vi "Display YAML in Tree.vi"(8 "error in (no error)":errorcluster, 10 "Tree Refnum":refnum<vi>, 11 "YAML Parser in":refnum<class "YAML Parser.lvclass">) -> (0 "error out":errorcluster, 3 "YAML Parser out":refnum<class "YAML Parser.lvclass">)   [LabVIEW 2015, in "YAML Parser.lvclass"]
uses:
  YAML Parser.lvclass
  YAML Parser.lvclass/YAML Parser.ctl
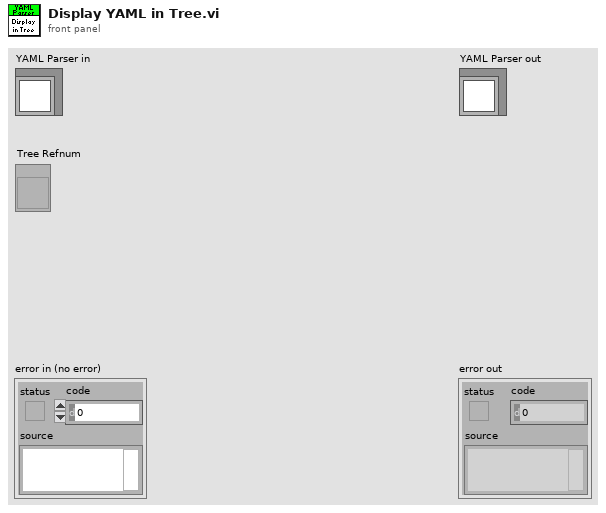
[diagram p1: front panel]
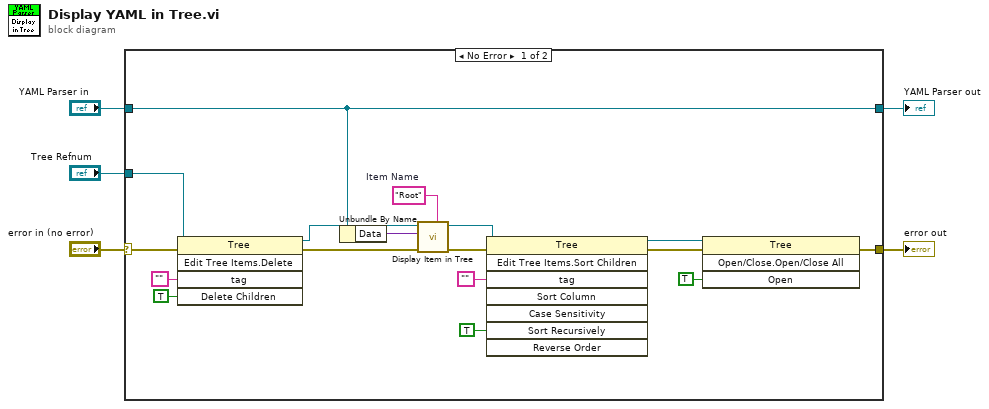
[diagram p0: block diagram]
diagram:
  n1 = case shown="No Error" "error in (no error)" {
    selector: "error in (no error)" -> [w22 w24]
    tunnel: [w11 w24] -> w4
    tunnel: [w18 w23] -> w2
    tunnel: "YAML Parser in" -> [w18 w23]
    tunnel: "Tree Refnum" -> [w21 _]
    frame No Error {
      w8 = "Root"  # Item Name
      n2 = invoke class="Tree" method="Edit Tree Items.Delete"(reference=w21, error in=w22, "tag"="", "Delete Children"=TRUE) -> (reference out=w15:refnum<vi>, error out=w17:errorcluster)  [unwired: 1 in, 3 out]
      n3 = Unbundle By Name(w18) -> ("Data"=w16:variant)
      n4 = call "Display Item in Tree.vi"("Item Name"=w8, "error in (no error)"=w17, "Data"=w16, "Tree Refnum"=w15) -> ("error out"=w14:errorcluster, "Tree Refnum out"=w10:refnum<vi>)  [unwired: 6 in]
      n5 = invoke class="Tree" method="Edit Tree Items.Sort Children"(reference=w10, error in=w14, "tag"="", "Sort Recursively"=TRUE) -> (reference out=w13:refnum<vi>, error out=w12:errorcluster)  [unwired: 4 in, 6 out]
      n6 = invoke class="Tree" method="Open/Close.Open/Close All"(reference=w13, error in=w12, "Open"=TRUE) -> (error out=w11:errorcluster)  [unwired: 1 in, 3 out]
    }
    frame Error {
    }
  }
  "error out" <- w4
  "YAML Parser out" <- w2
